vi "RANGE Mass Flow Unit Conversion.vi"(4 "Meter Units Out":T1, 7 "Ft³/HR -SLPM (T)":bool, 8 "Error In":errorcluster, 11 "Input Mass Flow Rate":dbl) -> (0 "Error Out":errorcluster, 3 "Output Mass Flow Rate":dbl)   [LabVIEW 2020]
uses:
  Drivers/Omega FMA-1600A Series Gas Flow Meter/Type Definitions/FMA1600A Units String.ctl
  Drivers/Alicat Gas Meter Driver/Sub-VIs/Units of Measure.ctl
panel:
  out "Ft³/HR":dbl
  out "SLPM":dbl
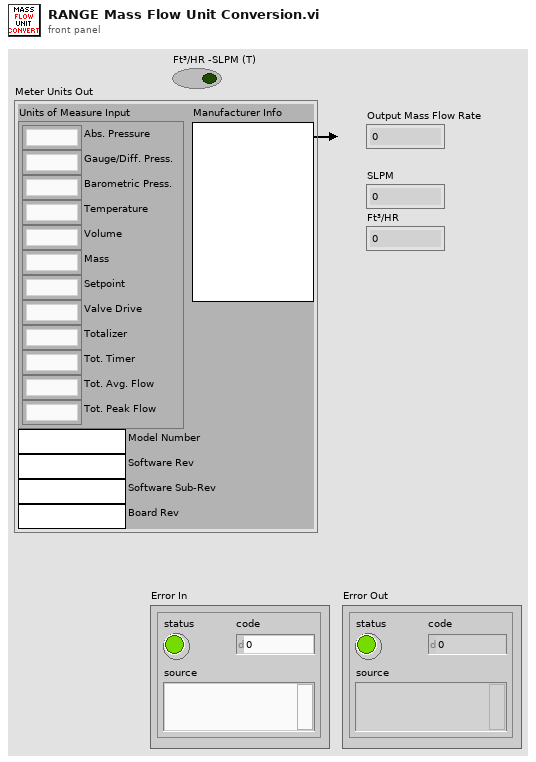
[diagram p1: front panel]
types:
  T1 = typedef "FMA1600A Units String.ctl" = cluster{"Software Rev":string, "Model Number":string, "Manufacturer Info":string, "Software Sub-Rev":string, "Board Rev":string, "Units of Measure Input":T2}
  T2 = typedef "Units of Measure.ctl" = cluster{"Abs. Pressure":string, "Gauge/Diff. Press.":string, "Barometric Press.":string, "Temperature":string, "Volume":string, "Mass":string, "Setpoint":string, "Valve Drive":string, "Totalizer":string, "Tot. Timer":string, "Tot. Avg. Flow":string, "Tot. Peak Flow":string}
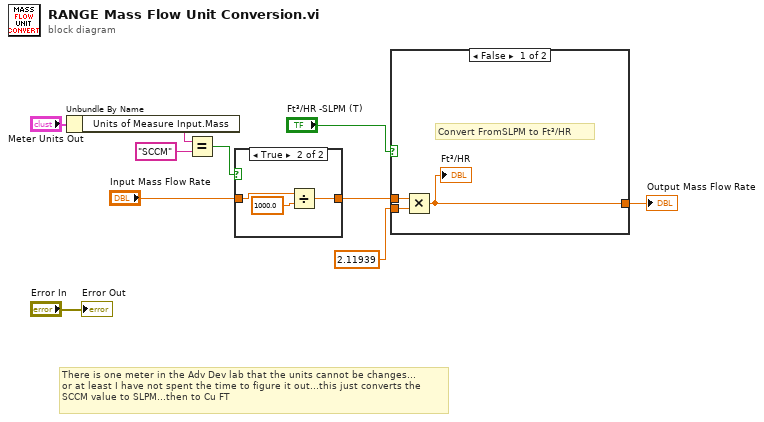
[diagram p0: block diagram]
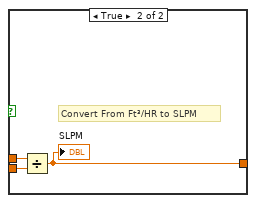
[diagram p3: hidden frame]
diagram:
  # "There is one meter in the Adv Dev lab that the units cannot be changes...\nor at least I have not spent the time to figure it out...this just converts the \nSCCM value to SLPM...then to Cu FT"
  n1 = Unbundle By Name("Meter Units Out") -> ("Units of Measure Input.Mass"=w5:string)
  n2 = Equal?(x=w5, y="SCCM") -> (x = y?=w3:bool)
  n3 = case shown="True" w3 {
    tunnel: "Input Mass Flow Rate" -> [w11 w14]
    tunnel: [w11 w12] -> w1
    frame False {
    }
    frame True {
      n4 = Divide(x=w14, y=1000.0) -> (x/y=w12:dbl)
    }
  }
  n5 = case shown="False" "Ft³/HR -SLPM (T)" {
    tunnel: w1 -> [w17 w20]
    tunnel: [w15 w19] -> w9
    tunnel: 2.11939 ("y") -> [w16 w18]
    frame False {
      # "Convert FromSLPM to Ft³/HR"
      n6 = Multiply(x=w17, y=w16) -> (x*y=w15:dbl)
      "Ft³/HR" <- w15
    }
    frame True {
      # "Convert From Ft³/HR to SLPM"
      n7 = Divide(x=w20, y=w18) -> (x/y=w19:dbl)
      "SLPM" <- w19
    }
  }
  "Output Mass Flow Rate" <- w9
  "Error Out" <- "Error In"
